vi "_Select.vi"(0 "stdout fd":u64 format="%016x", 1 "deadline":T1={"mode"=enum."Relative", "deadline (ms)"=30000}, 5 "stderr fd":u64 format="%016x", 7 "stdin fd":u64 format="%016x", 9 "read size":i32, 11 "error in (no error)":errorcluster, 12 "select stdin":bool, 13 "select stdout":bool, 14 "select stderr":bool) -> (2 "stderr eof?":bool, 3 "stdout eof?":bool, 4 "stdout data":u8[](array[numeric]), 6 "stderr data":u8[](array[numeric]), 8 "stdin ready?":bool, 15 "error out":errorcluster)   [LabVIEW 2020, in "NI_Subprocess.lvlib" / "Subprocess.lvclass"]
uses:
  <vilib>/Subprocess/Subprocess/Subprocess.lvclass
  <vilib>/Utility/Deadline/Deadline.ctl
  <vilib>/Utility/Deadline/Mode.ctl
  lviosrg.dll
  <vilib>/Utility/Deadline/NI_Deadline.lvlib
  <vilib>/ErrorRing/Error Ring.xnode
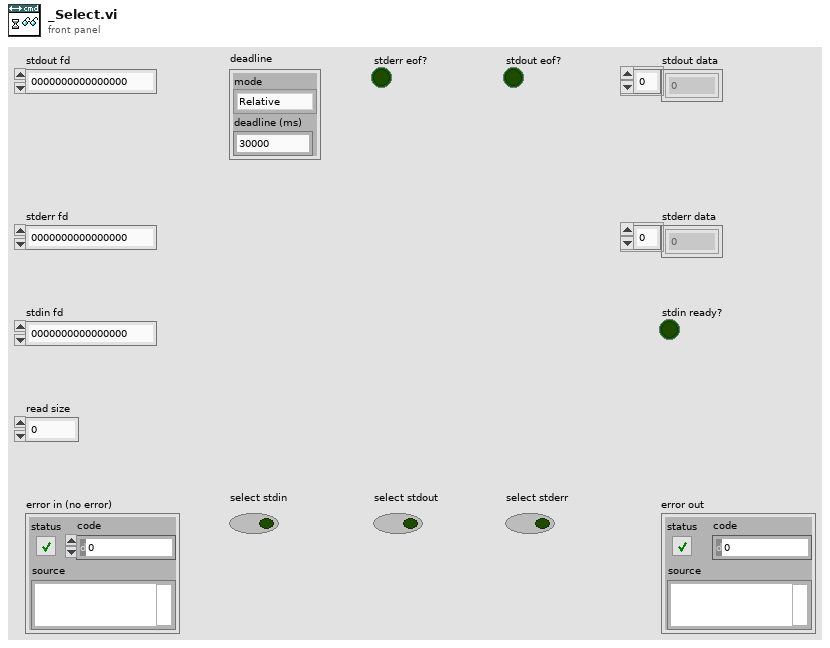
[diagram p1: front panel]
types:
  T1 = typedef "NI_Deadline.lvlib/Deadline.ctl" = cluster{"mode":T2, "deadline (ms)":u32}
  T2 = typedef "NI_Deadline.lvlib/Mode.ctl" = enum16{"Relative", "Use deadline", "Wait forever", "Nonblocking", "N/A"}
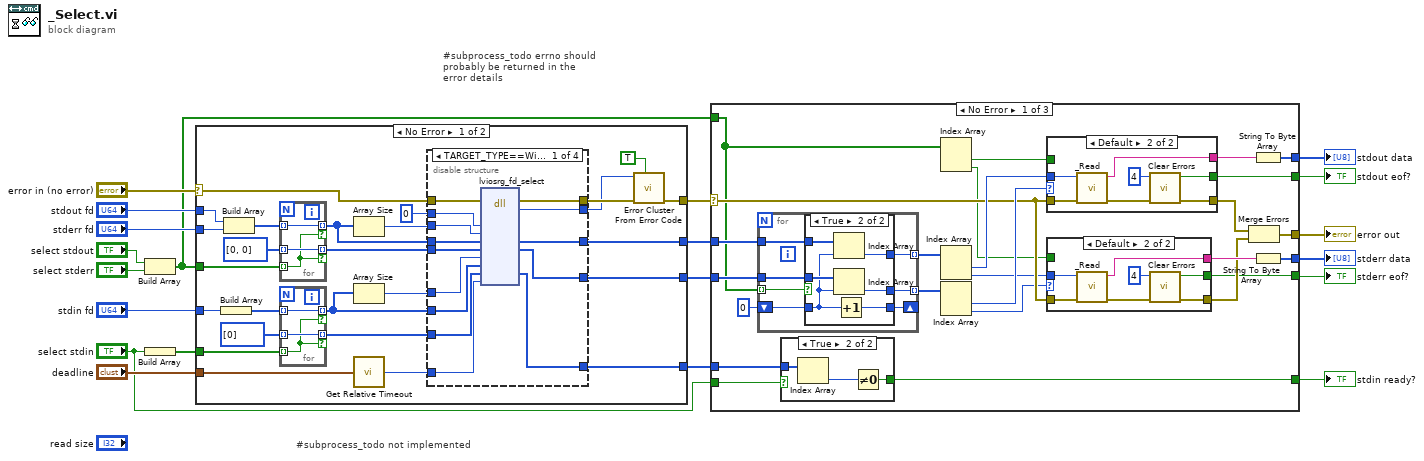
[diagram p0: block diagram]
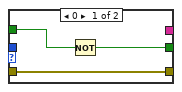
[diagram p4: hidden frame]
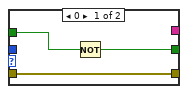
[diagram p5: hidden frame]
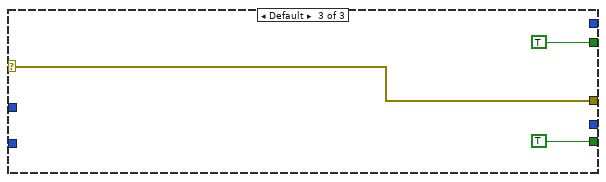
[diagram p7: hidden frame]
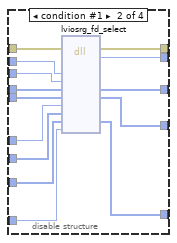
[diagram p8: hidden frame]
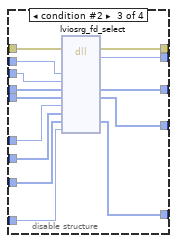
[diagram p9: hidden frame]
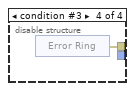
[diagram p10: hidden frame]
diagram:
  # "#subprocess_todo errno should probably be returned in the error details"
  # "#subprocess_todo not implemented"
  n1 = Build Array("select stdout", "select stderr") -> (w6:bool[])
  n2 = Build Array("select stdin") -> (w4:bool[])
  n3 = case shown="No Error" "error in (no error)" {
    selector: "error in (no error)" -> [w41 w100]
    tunnel: "stdout fd" -> [w38 _]
    tunnel: "stderr fd" -> [w37 _]
    tunnel: [w44 _] -> w12
    tunnel: [w22 w100] -> w10
    tunnel: [w43 _] -> w11
    tunnel: "deadline" -> [w40 _]
    tunnel: w6 -> [w35 _]
    tunnel: "stdin fd" -> [w29 _]
    tunnel: w4 -> [w28 _]
    tunnel: [w24 _] -> w2
    frame No Error {
      n4 = Build Array(w29) -> (w31:u64[])
      n5 = Build Array(w38, w37) -> (w36:u64[])
      n6 = for {
        tunnel: w35 -> [w97] mode=indexing
        tunnel: w36 -> [w99] mode=indexing
        tunnel: [w99] -> w34 mode=indexing if=w97
        tunnel: u8[] [0, 0] ("write_fds") -> [w98] mode=indexing
        tunnel: [w98] -> w32 mode=indexing if=w97
      }
      n7 = for {
        tunnel: w28 -> [w94] mode=indexing
        tunnel: w31 -> [w96] mode=indexing
        tunnel: [w96] -> w26 mode=indexing if=w94
        tunnel: u8[] [0] ("write_fds") -> [w95] mode=indexing
        tunnel: [w95] -> w25 mode=indexing if=w94
      }
      n8 = Array Size(array=w34) -> (size(s)=w45:i32)
      n9 = Array Size(array=w26) -> (size(s)=w27:i32)
      n10 = call <vilib>:"Get Relative Timeout.vi"("Timeout"=w40) -> ("timeout (ms) out"=w39:i32)
      n11 = disable-structure "Conditional Disable Structure" shown="TARGET_TYPE==Windows||OS==Win" {
        disable-tunnel: 0 ("errno") -> [w60 w74 w88 _]
        disable-tunnel: w34 -> [w59 w73 w78 _]
        disable-tunnel: w45 -> [w58 w72 w87 _]
        disable-tunnel: w27 -> [w57 w71 w86 _]
        disable-tunnel: w26 -> [w51 w63 w80 _]
        disable-tunnel: w39 -> [w56 w70 w85 _]
        disable-tunnel: [w49 w69 w84 _] -> w43
        disable-tunnel: [w50 w68 w83 _] -> w44
        disable-tunnel: [w55 w67 w82 w89] -> w42
        disable-tunnel: w41 -> [w54 w66 w81 _]
        disable-tunnel: [w53 w64 w79 _] -> w23
        disable-tunnel: w32 -> [w52 w65 w77 _]
        disable-tunnel: w25 -> [w48 w62 w76 _]
        disable-tunnel: [w47 w61 w75 _] -> w24
        frame condition #0 (active) {
          n12 = dll-call lib="lviosrg.*" fn="lviosrg_fd_select"(error in=w54, "errno"=w60, "readCnt"=w58, "read_fds"=w59, "read_fds_ready"=w52, "writeCnt"=w57, "write_fds"=w51, "write_fds_ready"=w48, "timeOut"=w56) -> (error out=w55:errorcluster, "return type"=w53:i32, "read_fds"=w50:u64[], "read_fds_ready"=w49:u8[], "write_fds_ready"=w47:i32[])  [unwired: 9 in, 1 out]
        }
        frame condition #1 {
          n13 = dll-call lib="lviosrg.*" fn="lviosrg_fd_select"(error in=w66, "errno"=w74, "readCnt"=w72, "read_fds"=w73, "read_fds_ready"=w65, "writeCnt"=w71, "write_fds"=w63, "write_fds_ready"=w62, "timeOut"=w70) -> (error out=w67:errorcluster, "return type"=w64:i32, "read_fds"=w68:u64[], "read_fds_ready"=w69:u8[], "write_fds_ready"=w61:i32[])  [unwired: 9 in, 1 out]
        }
        frame condition #2 {
          n14 = dll-call lib="lviosrg.*" fn="lviosrg_fd_select"(error in=w81, "errno"=w88, "readCnt"=w87, "read_fds"=w78, "read_fds_ready"=w77, "writeCnt"=w86, "write_fds"=w80, "write_fds_ready"=w76, "timeOut"=w85) -> (error out=w82:errorcluster, "return type"=w79:i32, "read_fds"=w83:u64[], "read_fds_ready"=w84:u8[], "write_fds_ready"=w75:i32[])  [unwired: 9 in, 1 out]
        }
        frame condition #3 {
          n15 = xnode ("Error Ring")() -> ("error out"=w89:errorcluster)
        }
      }
      n16 = call <vilib>:"Error Cluster From Error Code.vi"("show call chain? (False)"=TRUE, "error in (no error)"=w42, "error code (0)"=w23) -> ("error out"=w22:errorcluster)  [unwired: 6 in]
    }
    frame Error {
    }
  }
  n17 = case shown="No Error" w10 {
    selector: w10 -> [w122 w163 w166]
    tunnel: w12 -> [w111 _ _]
    tunnel: w11 -> [w110 _ _]
    tunnel: [w114 w163 w166] -> w14
    tunnel: [w125 _ _] -> w17
    tunnel: [w118 _ _] -> w18
    tunnel: [w113 _ TRUE] -> w15
    tunnel: [w101 _ TRUE] -> w16
    tunnel: w6 -> [w107 _ _]
    tunnel: "select stdin" -> [w104 _ _]
    tunnel: w2 -> [w103 _ _]
    tunnel: [w102 _ _] -> w1
    frame No Error {
      n18 = for {
        tunnel: w107 -> [w135] mode=indexing
        tunnel: w111 -> [w134]
        shift-right: [w132] -> _
        shift-left: 0 -> [w133]
        tunnel: [w131] -> w109 mode=indexing
        tunnel: w110 -> [w130]
        tunnel: [w129] -> w108 mode=indexing
        n19 = case shown="True" w135 {
          tunnel: w134 -> [_ w142]
          tunnel: w133 -> [w136 w137]
          tunnel: [w136 w141] -> w132
          tunnel: [_ w140] -> w131
          tunnel: w130 -> [_ w139]
          tunnel: [_ w138] -> w129
          frame False {
          }
          frame True {
            n20 = Index Array(array=w142, index=w137) -> (element=w140:u64)
            n21 = Index Array(array=w139, index=w137) -> (element=w138:u8)
            n22 = Increment(x=w137) -> (x+1=w141:i32)
          }
        }
      }
      n23 = case shown="True" w104 {
        tunnel: w103 -> [_ w128]
        tunnel: [_ w126] -> w102
        frame False {
        }
        frame True {
          n24 = Index Array(array=w128) -> (element=w127:i32)  [unwired: 1 in]
          n25 = Not Equal To 0?(x=w127) -> (x != 0?=w126:bool)
        }
      }
      n26 = Index Array(array=w107) -> (element #1=w105:bool, element #2=w106:bool)  [unwired: 2 in]
      n27 = Index Array(array=w109) -> (element #1=w124:u64, element #2=w121:u64)  [unwired: 2 in]
      n28 = Index Array(array=w108) -> (element #1=w123:u8, element #2=w120:u8)  [unwired: 2 in]
      n29 = case shown="Default" w123 {
        tunnel: w124 -> [_ w162]
        tunnel: w122 -> [w155 w161]
        tunnel: [w155 w156] -> w116
        tunnel: [_ w160] -> w119
        tunnel: [w153 w157] -> w101
        tunnel: w105 -> [w154 _]
        frame 0 {
          n30 = Not(x=w154) -> (.not. x?=w153:bool)
        }
        frame Default {
          n31 = call <vilib>:"_Read.vi"("error in"=w161, "fd"=w162) -> ("error out"=w159:errorcluster, "buf"=w160:string)  [unwired: 7 in, 1 out]
          n32 = call <vilib>:"Clear Errors.vi"("error in (no error)"=w159, "specific error code to clear (0: all)"=4) -> ("error out"=w156:errorcluster, "specific error cleared?"=w157:bool)  [unwired: 4 in]
        }
      }
      n33 = case shown="Default" w120 {
        tunnel: w121 -> [_ w152]
        tunnel: w122 -> [w145 w151]
        tunnel: [w145 w149] -> w115
        tunnel: [_ w147] -> w117
        tunnel: [w143 w146] -> w113
        tunnel: w106 -> [w144 _]
        frame 0 {
          n34 = Not(x=w144) -> (.not. x?=w143:bool)
        }
        frame Default {
          n35 = call <vilib>:"_Read.vi"("error in"=w151, "fd"=w152) -> ("error out"=w148:errorcluster, "buf"=w147:string)  [unwired: 7 in, 1 out]
          n36 = call <vilib>:"Clear Errors.vi"("error in (no error)"=w148, "specific error code to clear (0: all)"=4) -> ("error out"=w149:errorcluster, "specific error cleared?"=w146:bool)  [unwired: 4 in]
        }
      }
      n37 = Merge Errors(w116, w115) -> (w114:errorcluster)
      n38 = String To Byte Array(string=w119) -> (unsigned byte array=w118:u8[])
      n39 = String To Byte Array(string=w117) -> (unsigned byte array=w125:u8[])
    }
    frame Error {
    }
    frame Default {
    }
  }
  "error out" <- w14
  "stdout eof?" <- w16
  "stdout data" <- w18
  "stderr data" <- w17
  "stderr eof?" <- w15
  "stdin ready?" <- w1
